vi "Autonomous Independent.vi"() -> ()   [LabVIEW 2014]
doc: "This VI is called when autonomous begins, and will automatically be terminated when autonomous ends. You can carry out timed or sensor driven robot movement independently without needing to return to the caller."
uses:
  <vilib>/Rock Robotics/WPI/Joystick/WPI_JoystickGetSetRefNum.vi
  Robot Global Data.vi
  <vilib>/Rock Robotics/WPI/RobotDrive/WPI_RobotDriveGetSetRefNum.vi
  <vilib>/Rock Robotics/WPI/RobotDrive/WPI_RobotDriveMecanumDrive_Cartesian.vi
panel:
  in  "How many totes are we picking up":dbl
  in  "iteration":dbl
  in  "time after tote lifted":dbl
  in  "lifter state machine auton":T1(ring)
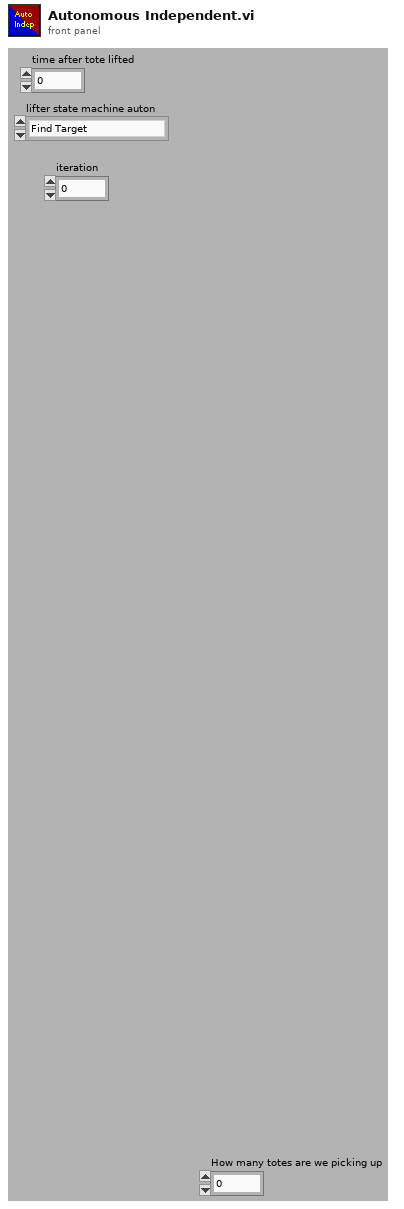
[diagram p1: front panel]
types:
  T1 = enum16{"Find Target", "Move to target", "Lower tote", "Pick up tote", "Back up", "Move foward", "Put totes down"}
  T2 = cluster{"Total Center of Mass":cluster{"X":dbl, "Y":dbl}, "average distance":dbl}
  T3 = typedef "WPI_UltrasonicDeviceRef.ctl" = cluster{"DevStatus":errorcluster, "Ping Digital Module":T4, "Echo Digital Module":T4, "Ping Channel":T5, "Echo Channel":T5, "CntIndex":T6}
  T4 = typedef "FPGA_TypedefDigitalModule.ctl" = enum16{"Digital Module 1", "Digital Module 2"}
  T5 = typedef "FPGA_DIOChannel.ctl" = enum8{"DIO 1", "DIO 2", "DIO 3", "DIO 4", "DIO 5", "DIO 6", "DIO 7", "DIO 8", "DIO 9", "DIO 10", "DIO 11", "DIO 12", "DIO 13", "DIO 14", "Invalid"}
  T6 = typedef "FPGA_CounterCtrSystemIndex.ctl" = enum8{"Ctr 0", "Ctr 1", "Ctr 2", "Ctr 3", "Ctr 4", "Ctr 5", "Ctr 6", "Ctr 7", "Invalid"}
  T7 = typedef "WPI_JoystickDevRef.ctl" = cluster{"Device":T8}
  T8 = typedef "WPI_JoystickDeviceEnum.ctl" = enum16{"USB 0", "USB 1", "USB 2", "USB 3", "USB 4", "USB 5"}
  T9 = typedef "Joystick Buttons typedef.ctl" = cluster{"A":bool, "B":bool, "X":bool, "Y":bool, "Left bumper":bool, "Right bumper":bool, "Select":bool, "Start":bool}
  T10 = typedef "WPI_MotorControlDeviceRef.ctl" = cluster{"DeviceStatus":errorcluster, "Type":enum16{"PWM", "CAN"}, "PWM":cluster{"Digital Module":T4, "PWM Channel":T11, "DeadBand":T12}, "CAN":cluster{"Device Number":u8, "Control Mode":T13, "Semaphore":T14, "Max Vout":dbl}, "Invert":bool, "TransformRef":T15, "InvTransformRef":T15}
  T11 = typedef "FPGA_DIOPWMChannel.ctl" = enum8{"PWM 1", "PWM 2", "PWM 3", "PWM 4", "PWM 5", "PWM 6", "PWM 7", "PWM 8", "PWM 9", "PWM 10", "Invalid"}
  T12 = typedef "WPI_PWMDeadband.ctl" = cluster{"Name":string, "maxPositivePwm":i32, "minPositivePwm":i32, "centerPwm":i32, "maxNegativePwm":i32, "minNegativePwm":i32, "angularRange":u16}
  T13 = typedef "WPI_CANJaguar_ControlMode.ctl" = enum8{"Percent VBus", "Current", "Speed", "Position", "Voltage"}
  T14 = typedef "Semaphore RefNum" = refnum<k1>
  T15 = typedef "WPI_PWMTransform_ConPane.ctl" = refnum<vi>
  T16 = typedef "WPI_RobotDriveDevRef.ctl" = cluster{"DevStatus":errorcluster, "Motors[]":T10[], "Square Inputs":bool, "Max Output":dbl}
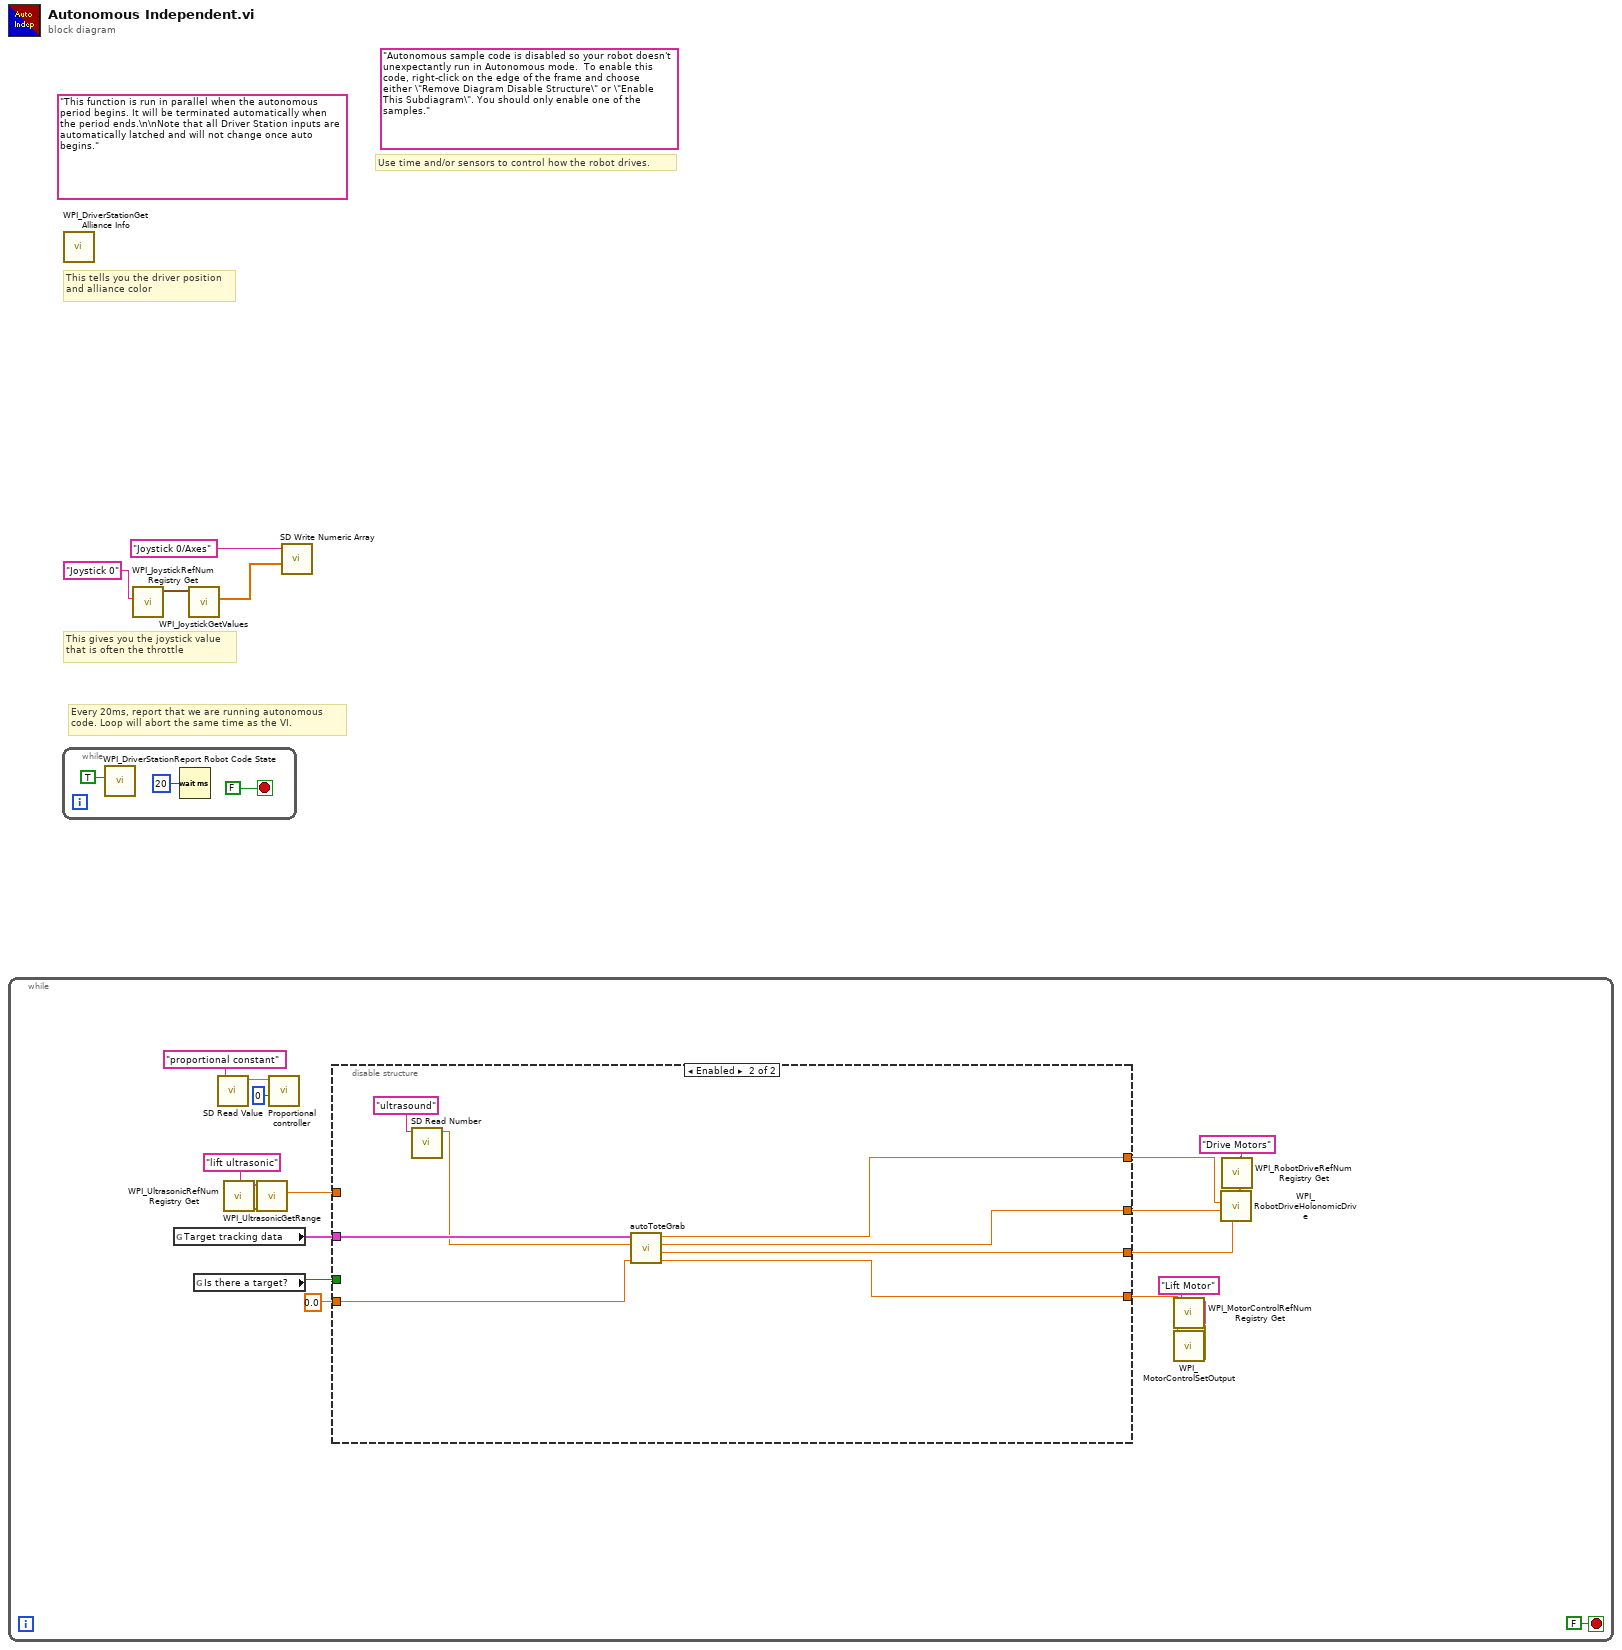
[diagram p0: block diagram]
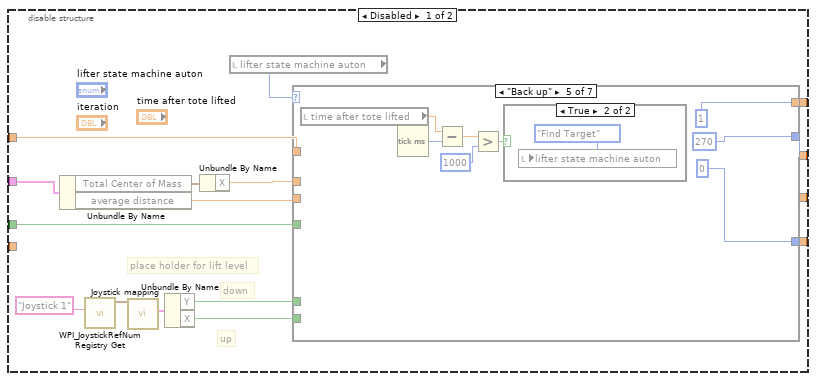
[diagram p2: hidden frame]
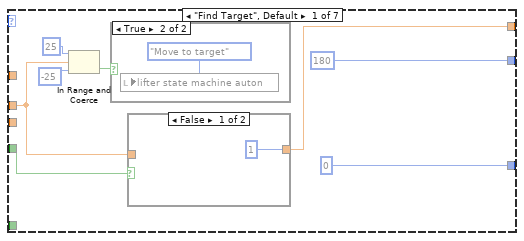
[diagram p3: hidden frame]
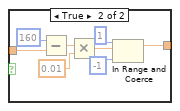
[diagram p4: hidden frame]
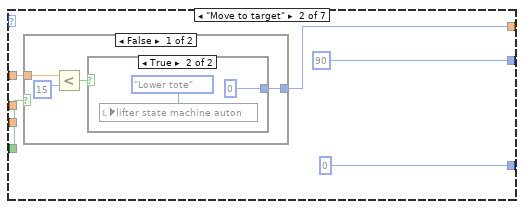
[diagram p6: hidden frame]
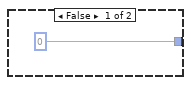
[diagram p7: hidden frame]
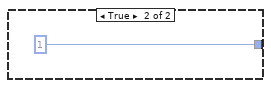
[diagram p8: hidden frame]
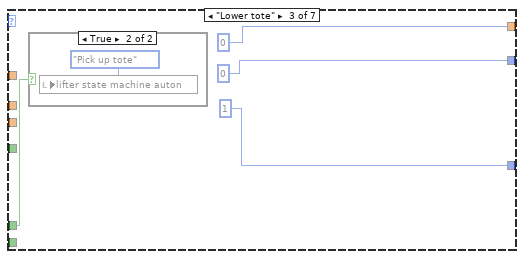
[diagram p9: hidden frame]
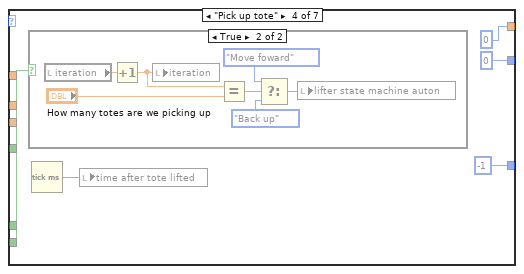
[diagram p11: hidden frame]
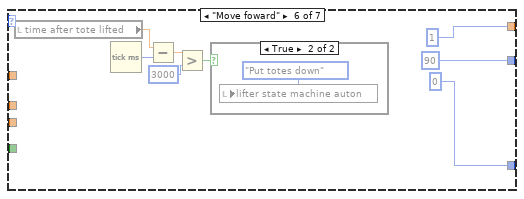
[diagram p14: hidden frame]
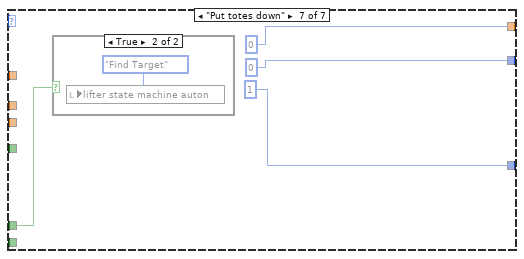
[diagram p16: hidden frame]
diagram:
  (unwired) "Autonomous sample code is disabled so your robot doesn't unexpectantly run in Autonomous mode.  To enable this code, right-click on the edge of the frame and choose either \"Remove Diagram Disable Structure\" or \"Enable This Subdiagram\". You should only enable one of the samples."
  (unwired) "This function is run in parallel when the autonomous period begins. It will be terminated automatically when the period ends.\n\nNote that all Driver Station inputs are automatically latched and will not change once auto begins."
  # "Every 20ms, report that we are running autonomous\ncode. Loop will abort the same time as the VI."
  # "This gives you the joystick value\nthat is often the throttle"
  # "Use time and/or sensors to control how the robot drives."
  # "This tells you the driver position\nand alliance color"
  n1 = while {
    stop <- FALSE stop-if-true
    n2 = global read "Robot Global Data.vi" "Target tracking data"() -> (w8:T2)
    n3 = global read "Robot Global Data.vi" "Is there a target?"() -> (w19:bool)
    n4 = call-poly <vilib>:"SD Read Value.vi"("Table Prefix"="proportional constant") -> ("Numeric"=w20:dbl)  [unwired: 8 in, 2 out]
    n5 = call <vilib>:"WPI_UltrasonicRefNum Registry Get.vi"("refnum name"="lift ultrasonic") -> ("error out"=w17:errorcluster, "UltrasonicDevRef"=w11:T3)  [unwired: 9 in]
    n6 = call <vilib>:"WPI_UltrasonicGetRange.vi"("error in (no error)"=w17, "UltrasonicDevRef"=w11) -> ("Distance"=w16:dbl)  [unwired: 7 in, 2 out]
    n7 = call "Proportional controller.vi"("setpoint"=0, "proportional control"=w20) -> ()  [unwired: 9 in, 1 out]
    n8 = disable-structure shown="Enabled" {
      disable-tunnel: [w38 w116] -> w22
      disable-tunnel: w8 -> [w25 w118]
      disable-tunnel: w19 -> [w37 _]
      disable-tunnel: w16 -> [w36 _]
      disable-tunnel: [w35 w113] -> w12
      disable-tunnel: [w29 w115] -> w10
      disable-tunnel: 0.0 -> [_ w117]
      disable-tunnel: [_ w114] -> w7
      frame Disabled {
        # "down"
        # "up"
        # "place holder for lift level"
        n9 = Unbundle By Name(w25) -> ("Total Center of Mass"=w28:cluster{"X":dbl, "Y":dbl}, "average distance"=w26:dbl)
        n10 = call <vilib>:"WPI_JoystickRefNum Registry Get.vi"("refnum name"="Joystick 1") -> ("JoystickDevRef"=w33:T7)  [unwired: 9 in, 1 out]
        n11 = call "Joystick mapping.vi"("JoystickDevRef"=w33) -> ("Joystick Buttons"=w32:T9)  [unwired: 9 in, 1 out]
        n12 = Unbundle By Name(w32) -> ("Y"=w31:bool, "X"=w30:bool)
        n13 = Unbundle By Name(w28) -> ("X"=w27:dbl)
        n14 = local read "lifter state machine auton"() -> (w39:T1)
        n15 = case shown="\"Back up\"" w39 {
          tunnel: [180 90 0 0 270 90 0] -> w29
          tunnel: [w41 w60 0 0 1 1 0] -> w38
          tunnel: w27 -> [w40 _ _ _ _ _ _]
          tunnel: w37 -> [w42 w61 _ _ _ _ _]
          tunnel: w36 -> [_ w59 _ _ _ _ _]
          tunnel: [0 0 1 -1 0 0 1] -> w35
          tunnel: w31 -> [_ _ w73 _ _ _ w108]
          tunnel: w30 -> [_ _ _ w76 _ _ _]
          tunnel: w26 -> [_ _ _ _ _ _ _]
          frame "Find Target", Default {
            n16 = In Range and Coerce(upper limit=25, x=w40, lower limit=-25) -> (In Range?=w43:bool)  [unwired: 1 out]
            n17 = case shown="True" w43 {
              frame False {
              }
              frame True {
                n18 = local write "lifter state machine auton"(T1."Move to target" ("lifter state machine")) -> ()
              }
            }
            n19 = case shown="False" w42 {
              tunnel: [1 w49] -> w41
              tunnel: w40 -> [_ w55]
              frame False {
              }
              frame True {
                n20 = Subtract(x=160, y=w55) -> (x-y=w54:dbl)
                n21 = Multiply(x=w54, y=0.01) -> (x*y=w52:dbl)
                n22 = In Range and Coerce(upper limit=1, x=w52, lower limit=-1) -> (coerced(x)=w49:dbl)  [unwired: 1 out]
              }
            }
          }
          frame "Move to target" {
            n23 = case shown="False" w61 {
              tunnel: [w64 1] -> w60
              tunnel: w59 -> [w63 _]
              frame False {
                n24 = Less?(x=w63, y=15) -> (x < y?=w66:bool)
                n25 = case shown="True" w66 {
                  tunnel: [0 0] -> w64
                  frame False {
                  }
                  frame True {
                    n26 = local write "lifter state machine auton"(T1."Lower tote" ("lifter state machine")) -> ()
                  }
                }
              }
              frame True {
              }
            }
          }
          frame "Lower tote" {
            n27 = case shown="True" w73 {
              frame False {
              }
              frame True {
                n28 = local write "lifter state machine auton"(T1."Pick up tote" ("lifter state machine")) -> ()
              }
            }
          }
          frame "Pick up tote" {
            n29 = case shown="True" w76 {
              frame False {
              }
              frame True {
                n30 = local read "iteration"() -> (w87:dbl)
                n31 = Increment(x=w87) -> (x+1=w82:dbl)
                n32 = local write "iteration"(w82) -> ()
                n33 = Equal?(x=w82, y="How many totes are we picking up") -> (x = y?=w83:bool)
                n34 = Select(t=T1."Move foward" ("lifter state machine"), s=w83, f=T1."Back up" ("lifter state machine")) -> (s? t:f=w86:T1)
                n35 = local write "lifter state machine auton"(w86) -> ()
              }
            }
            n36 = Tick Count (ms)() -> (millisecond timer value=w79:u32)
            n37 = local write "time after tote lifted"(w79) -> ()
          }
          frame "Back up" {
            n38 = local read "time after tote lifted"() -> (w92:dbl)
            n39 = Tick Count (ms)() -> (millisecond timer value=w93:u32)
            n40 = Subtract(x=w92, y=w93) -> (x-y=w91:dbl)
            n41 = Greater?(x=w91, y=1000) -> (0:w89:bool)
            n42 = case shown="True" w89 {
              frame False {
              }
              frame True {
                n43 = local write "lifter state machine auton"(T1."Find Target" ("lifter state machine")) -> ()
              }
            }
          }
          frame "Move foward" {
            n44 = local read "time after tote lifted"() -> (w104:dbl)
            n45 = Tick Count (ms)() -> (millisecond timer value=w103:u32)
            n46 = Subtract(x=w104, y=w103) -> (x-y=w100:dbl)
            n47 = Greater?(x=w100, y=3000) -> (0:w98:bool)
            n48 = case shown="True" w98 {
              frame False {
              }
              frame True {
                n49 = local write "lifter state machine auton"(T1."Put totes down" ("lifter state machine")) -> ()
              }
            }
          }
          frame "Put totes down" {
            n50 = case shown="True" w108 {
              frame False {
              }
              frame True {
                n51 = local write "lifter state machine auton"(T1."Find Target" ("lifter state machine")) -> ()
              }
            }
          }
        }
      }
      frame Enabled {
        n52 = call <vilib>:"SD Read Number.vi"("Name"="ultrasound") -> ("Numeric"=w112:dbl)  [unwired: 8 in, 2 out]
        n53 = call "autoToteGrab.vi"("potValue"=w117, "ultrasonic"=w112, "Target tracking data"=w118) -> ("liftMotorOut"=w113:dbl, "holonomicRot"=w114:dbl, "holonomicY"=w115:dbl, "holonomicX"=w116:dbl)  [unwired: 5 in]
      }
    }
    n54 = call <vilib>:"WPI_MotorControlRefNum Registry Get.vi"("refnum name"="Lift Motor") -> ("error out"=w14:errorcluster, "MotorControlDevRef"=w13:T10)  [unwired: 9 in]
    n55 = call <vilib>:"WPI_MotorControlSetOutput.vi"("error in (no error)"=w14, "Output"=w12, "MotorControlDevRef"=w13) -> ()  [unwired: 6 in, 3 out]
    n56 = call <vilib>:"WPI_RobotDriveRefNum Registry Get.vi"("refnum name"="Drive Motors") -> ("RobotDriveDevRef"=w23:T16)  [unwired: 9 in, 1 out]
    n57 = call-poly <vilib>:"WPI_RobotDriveHolonomicDrive.vi"("Rotation"=w7, "Y"=w10, "X"=w22, "RobotDriveDevRef"=w23) -> ()  [unwired: 5 in, 3 out]
  }
  n58 = while {
    stop <- FALSE stop-if-true
    n59 = call <vilib>:"WPI_DriverStationReport Robot Code State.vi"("Autonomous"=TRUE) -> ()  [unwired: 10 in, 1 out]
    n60 = Wait (ms)(milliseconds to wait=u32 20) -> ()  [unwired: 1 out]
  }
  n61 = call <vilib>:"WPI_DriverStationGet Alliance Info.vi"() -> ()  [unwired: 12 out]
  n62 = call <vilib>:"WPI_JoystickRefNum Registry Get.vi"("refnum name"="Joystick 0") -> ("JoystickDevRef"=w3:T7)  [unwired: 1 in, 9 out]
  n63 = call <vilib>:"WPI_JoystickGetValues.vi"("JoystickDevRef"=w3) -> ("Axes"=w1:dbl[])  [unwired: 6 in, 4 out]
  n64 = call <vilib>:"SD Write Numeric Array.vi"("Numeric Array"=w1, "Name"="Joystick 0/Axes") -> ()  [unwired: 8 in, 2 out]
